vi "InitAsListener.vi"(8 "error in (no error)":errorcluster, 10 "TCP Connection":refnum<class "TCP.lvclass">, 11 "TcpReader in":refnum<class "TcpReader.lvclass">) -> (0 "error out":errorcluster, 3 "TcpReader out":refnum<class "TcpReader.lvclass">)   [LabVIEW 2013, in "TcpReader.lvclass"]
doc: "Initialize the TCP/IP reader as a listener (server). The listener is given a valid TCP/IP connection at startup and will not reconnect if the connection fails"
uses:
  TcpReader.lvclass
  Interface/TCP/TCP/TCP.lvclass
  TcpReader.lvclass/TcpReader.ctl
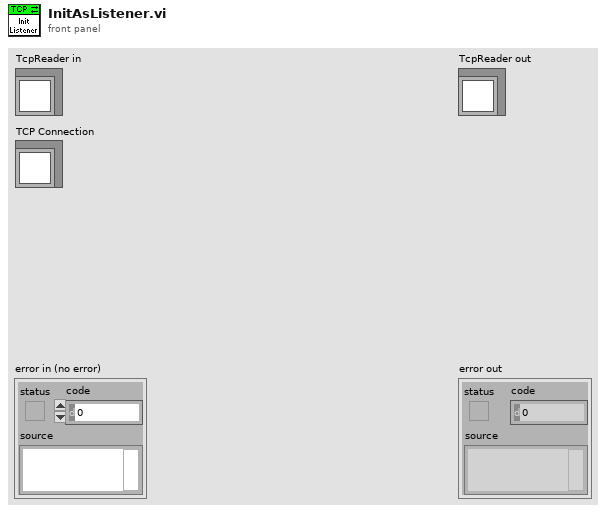
[diagram p1: front panel]
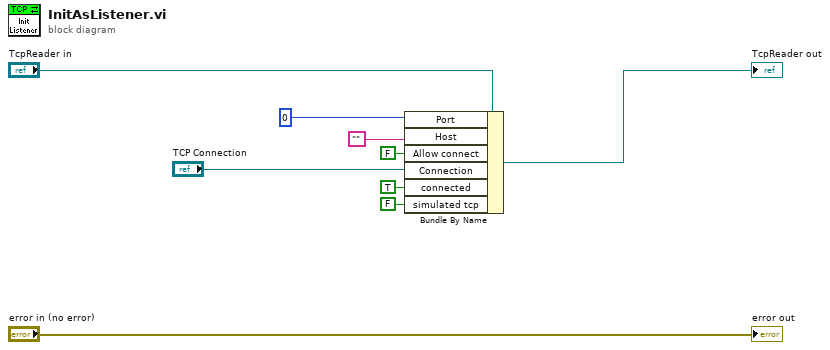
[diagram p0: block diagram]
diagram:
  n1 = Bundle By Name(cluster="TcpReader in", "Port"=u16 0 ("remote port"), "Host"="" ("address"), "Allow connect"=FALSE, "Connection"="TCP Connection", "connected"=TRUE, "simulated tcp"=FALSE) -> (→"TcpReader out":refnum<class "TcpReader.lvclass">)
  "error out" <- "error in (no error)"
